vi "Save Stats (Insert).vi"(0 "Filepath":path, 5 "Data":string[][](array[string]), 7 "DataRowIndex":i32, 9 "NumOfRows":i32, 11 "Error In":errorcluster) -> (4 "xlRefs":T1, 15 "Error Out":errorcluster)   [LabVIEW 2013]
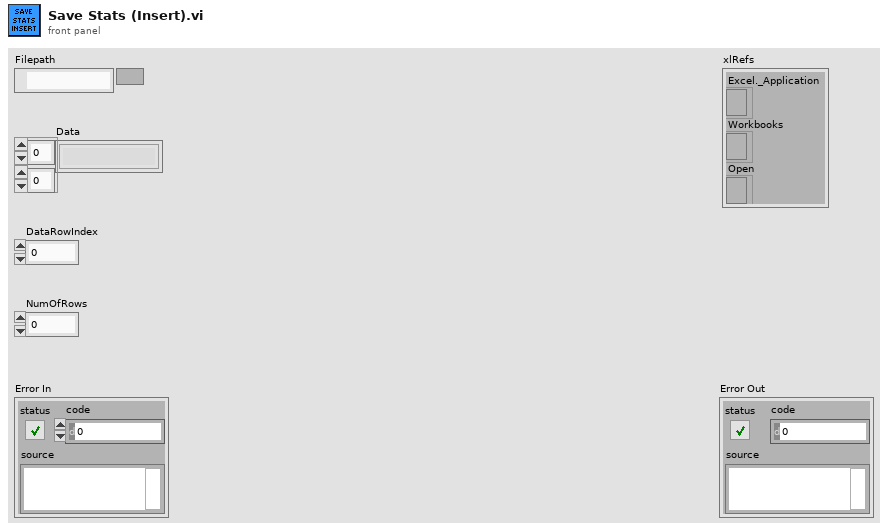
[diagram p1: front panel]
types:
  T1 = cluster{"Excel._Application":refnum<k7>, "Workbooks":refnum<k7>, "Open":refnum<k7>}
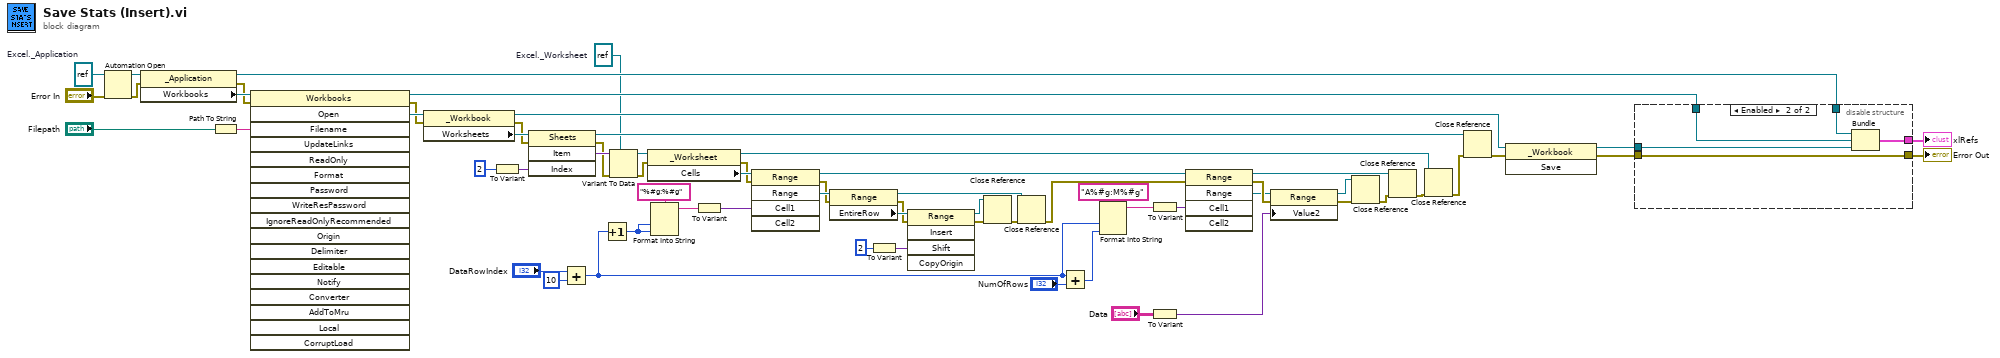
[diagram p0: block diagram]
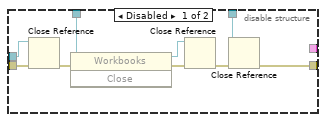
[diagram p2: hidden frame]
diagram:
  w49 = refnum<k7> refnum  # Excel._Worksheet
  w62 = refnum<k7> refnum  # Excel._Application
  n1 = Automation Open(error in (no error)="Error In", Automation Refnum=w62) -> (Automation Refnum=w63:refnum<k7>, error out=w64:errorcluster)  [unwired: 2 in]
  n2 = property class="_Application"(reference=w63, error in=w64) -> (reference out=w58:refnum<k7>, error out=w59:errorcluster, "Workbooks"=w65:refnum<k7>)
  n3 = Path To String(path="Filepath") -> (string=w55:string)
  n4 = invoke class="Workbooks" method="Open"(reference=w65, error in=w59, "Filename"=w55) -> (reference out=w60:refnum<k7>, error out=w57:errorcluster, "Open"=w61:refnum<k7>)  [unwired: 15 in, 15 out]
  n5 = property class="_Workbook"(reference=w61, error in=w57) -> (reference out=w52:refnum<k7>, error out=w28:errorcluster, "Worksheets"=w29:refnum<k7>)
  n6 = To Variant(anything=2) -> (Variant=w44:variant)
  n7 = invoke class="Sheets" method="Item"(reference=w29, error in=w28, "Index"=w44) -> (reference out=w50:refnum<k7>, error out=w42:errorcluster, "Item"=w43:variant)  [unwired: 1 in, 1 out]
  n8 = Add(x="DataRowIndex", y=10) -> (x+y=w3:i32)
  n9 = Increment(x=w3) -> (x+1=w2:i32)
  n10 = Variant To Data(error in=w42, type=w49, Variant=w43) -> (data=w26:refnum<k7>, error out=w25:errorcluster)
  n11 = property class="_Worksheet"(reference=w26, error in=w25) -> (reference out=w40:refnum<k7>, error out=w7:errorcluster, "Cells"=w15:refnum<k7>)
  n12 = Format Into String(format string="%#g:%#g", w2, w2) -> (resulting string=w20:string)  [unwired: 2 in, 1 out]
  n13 = To Variant(anything=w20) -> (Variant=w16:variant)
  n14 = invoke class="Range" method="Range"(reference=w15, error in=w7, "Cell1"=w16) -> (reference out=w14:refnum<k7>, error out=w13:errorcluster, "Range"=w24:refnum<k7>)  [unwired: 2 in, 2 out]
  n15 = property class="Range"(reference=w24, error in=w13) -> (reference out=w8:refnum<k7>, error out=w12:errorcluster, "EntireRow"=w23:refnum<k7>)
  n16 = To Variant(anything=2) -> (Variant=w21:variant)
  n17 = invoke class="Range" method="Insert"(reference=w23, error in=w12, "Shift"=w21) -> (reference out=w9:refnum<k7>, error out=w11:errorcluster)  [unwired: 2 in, 3 out]
  n18 = Close Reference(reference=w9, error in (no error)=w11) -> (error out=w10:errorcluster)
  n19 = Close Reference(reference=w8, error in (no error)=w10) -> (error out=w6:errorcluster)
  n20 = Add(x=w3, y="NumOfRows") -> (x+y=w27:i32)
  n21 = Format Into String(format string="A%#g:M%#g", w3, w27) -> (resulting string=w31:string)  [unwired: 2 in, 1 out]
  n22 = To Variant(anything=w31) -> (Variant=w36:variant)
  n23 = To Variant(anything="Data") -> (Variant=w34:variant)
  n24 = invoke class="Range" method="Range"(reference=w14, error in=w6, "Cell1"=w36) -> (reference out=w39:refnum<k7>, error out=w35:errorcluster, "Range"=w30:refnum<k7>)  [unwired: 2 in, 2 out]
  n25 = property class="Range"(reference=w30, error in=w35, "Value2"=w34) -> (reference out=w33:refnum<k7>, error out=w32:errorcluster)
  n26 = Close Reference(reference=w33, error in (no error)=w32) -> (error out=w38:errorcluster)
  n27 = Close Reference(reference=w39, error in (no error)=w38) -> (error out=w41:errorcluster)
  n28 = Close Reference(reference=w40, error in (no error)=w41) -> (error out=w51:errorcluster)
  n29 = Close Reference(reference=w50, error in (no error)=w51) -> (error out=w56:errorcluster)
  n30 = invoke class="_Workbook" method="Save"(reference=w52, error in=w56) -> (reference out=w53:refnum<k7>, error out=w54:errorcluster)  [unwired: 1 in, 1 out]
  n31 = disable-structure shown="Enabled" {
    disable-tunnel: w60 -> [w73 w77]
    disable-tunnel: w58 -> [w70 w76]
    disable-tunnel: w54 -> [w68 w79]
    disable-tunnel: w53 -> [w67 w78]
    disable-tunnel: [w66 w79] -> w48
    disable-tunnel: [_ w75] -> w1
    frame Disabled {
      n32 = Close Reference(reference=w67, error in (no error)=w68) -> (error out=w69:errorcluster)
      n33 = invoke class="Workbooks" method="Close"(reference=w73, error in=w69) -> (reference out=w72:refnum<k7>, error out=w71:errorcluster)  [unwired: 1 in, 1 out]
      n34 = Close Reference(reference=w72, error in (no error)=w71) -> (error out=w74:errorcluster)
      n35 = Close Reference(reference=w70, error in (no error)=w74) -> (error out=w66:errorcluster)
    }
    frame Enabled {
      n36 = Bundle("Excel._Application"=w76, "Workbooks"=w77, "Open"=w78) -> (w75:T1)  [unwired: 1 in]
    }
  }
  "Error Out" <- w48
  "xlRefs" <- w1
